vi "ProducerConsumerStyle VI.vi"() -> ()   [LabVIEW 2023]
doc: "Use this template to build a producer/consumer design pattern. Use this template when you need to execute a process, such as data analysis, when a data source, such as a triggered acquisition, produces data at an uneven rate and you need to execute the process when the data becomes available."
uses:
  <vilib>/express/express shared/transition.llb/Dynamic To Waveform Array.vi
  <vilib>/express/express signal manip/GetorSetDDTAttributes/Set DDT Attributes/SetT0.vi
  <vilib>/express/express shared/transition.llb/Waveform Array To Dynamic.vi
  <vilib>/FPGAPlugInAG/USB-7856R OEM/niLvFpga_Open_USB-7856R OEM.vi
  <vilib>/rvi/interface/common/dynamic/niFpgaDynamicAddResources.vi
  <vilib>/rvi/interface/common/niFpgaWaitOnOcc.vi
  <vilib>/Utility/error.llb/Error Cluster From Error Code.vi
  <vilib>/FPGAPlugInAG/Dynamic/niLvFpga_Run_Dynamic.vi
  <vilib>/rvi/errors/niLvFpgaAdjustHostInterfaceError.vi
  <vilib>/FPGAPlugInAG/Dynamic/niLvFpga_Close_Dynamic.vi
  <vilib>/express/express signal manip/GetorSetDDTAttributes/Set DDT Attributes/Set DDT Properties.xnode
  <vilib>/rvi/interface/nirviOpenFPGA/nirviOpenFPGA.xnode
  FPGA Bitfiles/wip_FPGATarget_FPGAVIwithRMS_sDE+ysAwCS4.lvbitx
  FPGA VI with RMS.vi
  <vilib>/rvi/interface/nirviMethod/nirviMethod.xnode
  <vilib>/rvi/interface/nirviReadWriteControl/nirviReadWriteControl.xnode
  <vilib>/rvi/interface/nirviCloseFPGA/nirviCloseFPGA.xnode
  <vilib>/rvi/errors/niLvFpgaMergeErrorWithErrorCode.vi
  <vilib>/FPGAPlugInAG/Dynamic/niLvFpga_ConfigureFifo_Dynamic.vi
  <vilib>/FPGAPlugInAG/Dynamic/niLvFpga_StartFifo_Dynamic.vi
  NiFpgaLv.dll
  <vilib>/rvi/interface/Simulation/niFpgaSimulationCallBeginRW.vi
  <vilib>/FPGAPlugInAG/Dynamic/niLvFpga_ReadFifo_Dynamic.vi
panel:
  out "In Loop timed out?":bool
  out "Saving Data":bool
  in  "Stop Writing Data":bool
  in  "Number of Elements":u32=500
  in  "Count(Ticks)":u32
  out "Elements Remaining":u32
  out "Timed Out?":bool
  out "Loop TIme":u32
  out "Waveform Chart":sgl[](graph)
  out "Actual Depth":u32
  in  "Ending frequency":dbl=32770.0
  in  "Starting frequency":dbl=32750.0
  out "Number of steps":dbl=nan
  out "I/P Frequency Value":dbl
  in  "Step Value":dbl=1.0
  in  "stop":bool
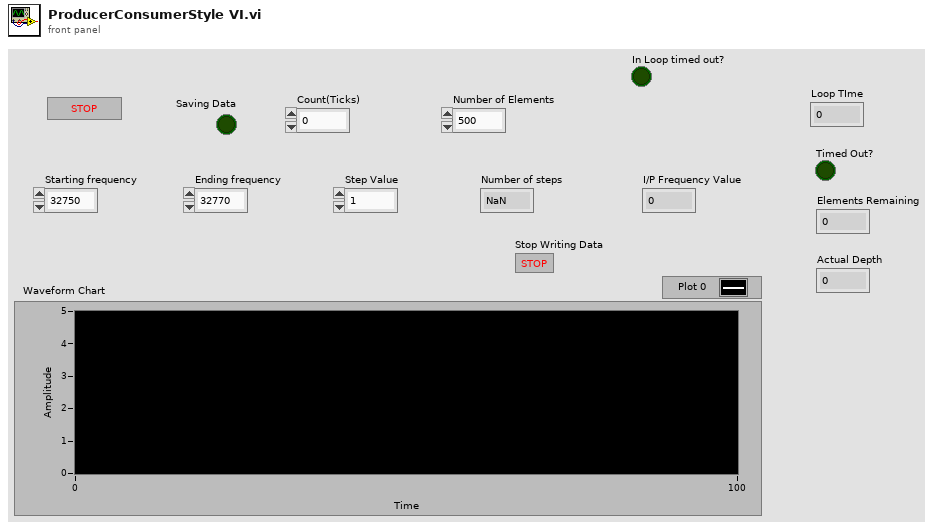
[diagram p1: front panel]
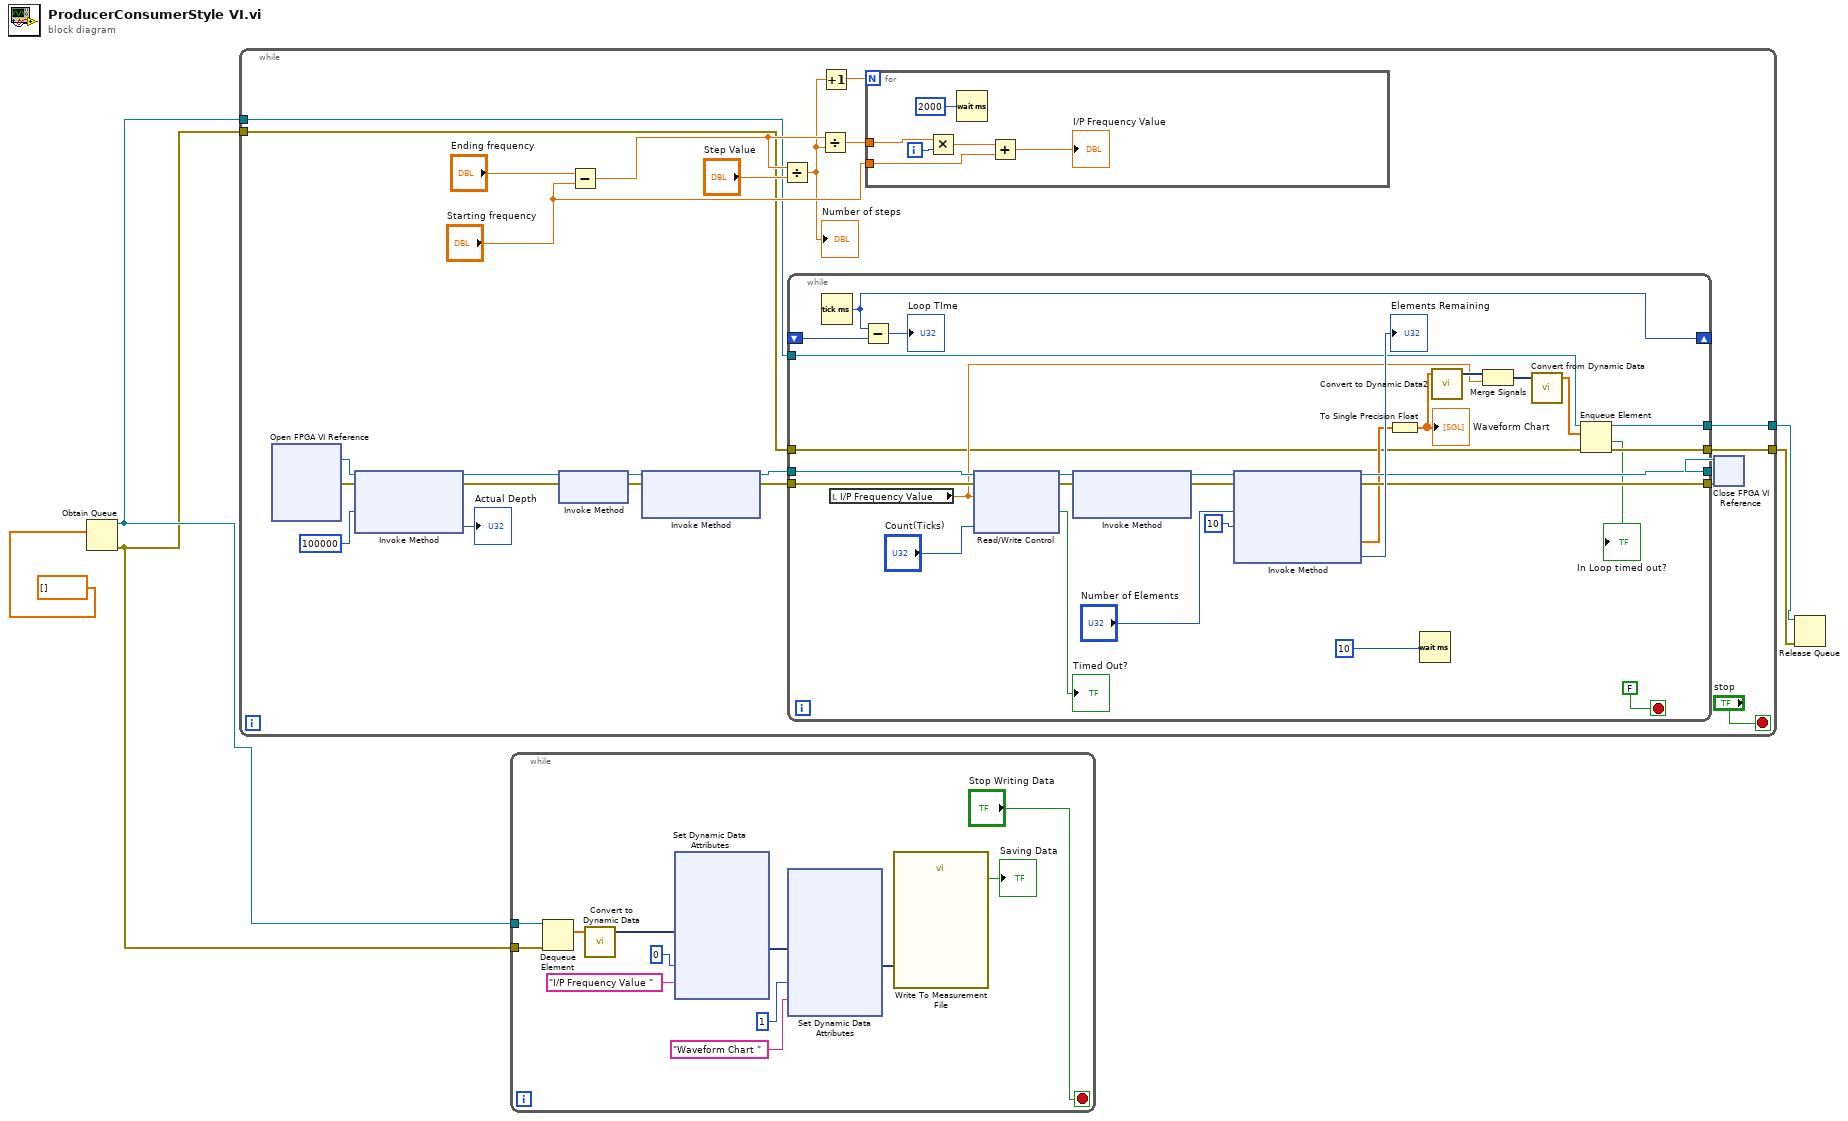
[diagram p0: block diagram]
diagram:
  n1 = Obtain Queue(element data type=dbl[] []) -> (queue out=w2:refnum<queue>, error out=w1:errorcluster)  [unwired: 4 in, 1 out]
  n2 = while {
    tunnel: [w9] -> w5
    tunnel: [w8] -> w4
    tunnel: w2 -> [w7]
    tunnel: w1 -> [w6]
    stop <- "stop" stop-if-true
    n3 = xnode "Open FPGA VI Reference"() -> ("FPGA VI Reference Out"=w28:refnum<k20>, "error out"=w27:errorcluster)  [unwired: 2 in]
    n4 = xnode "Invoke Method"("FPGA VI Reference In"=w28, "error in"=w27, "Requested Depth"=u32 100000) -> ("FPGA VI Reference Out"=w25:refnum<k20>, "error out"=w24:errorcluster, "Actual Depth"=→"Actual Depth":u32)
    n5 = xnode "Invoke Method"("FPGA VI Reference In"=w25, "error in"=w24) -> ("FPGA VI Reference Out"=w20:refnum<k20>, "error out"=w19:errorcluster)
    n6 = Subtract(x="Ending frequency", y="Starting frequency") -> (x-y=w12:dbl)
    n7 = xnode "Invoke Method"("FPGA VI Reference In"=w20, "error in"=w19) -> ("FPGA VI Reference Out"=w17:refnum<k20>, "error out"=w18:errorcluster)  [unwired: 1 in]
    n8 = Divide(x=w12, y="Step Value") -> (x/y=w10:dbl)
    "Number of steps" <- w10
    n9 = while {
      tunnel: [w62] -> w23
      tunnel: [w59] -> w22
      tunnel: w17 -> [w56]
      tunnel: w18 -> [w55]
      shift-right: [w51] -> _
      shift-left: _ -> [w50]
      tunnel: [w41] -> w9
      tunnel: [w40] -> w8
      tunnel: w7 -> [w39]
      tunnel: w6 -> [w38]
      stop <- FALSE stop-if-true
      n10 = Tick Count (ms)() -> (millisecond timer value=w51:u32)
      n11 = local read "I/P Frequency Value"() -> (w45:dbl)
      n12 = Subtract(x=w51, y=w50) -> (x-y=→"Loop TIme":u32)
      n13 = xnode "Read/Write Control"("FPGA VI Reference In"=w56, "error in"=w55, "Frequency"=w45, "Count(Ticks)"="Count(Ticks)") -> ("FPGA VI Reference Out"=w54:refnum<k20>, "error out"=w53:errorcluster, "Timed Out?"=→"Timed Out?":bool)
      n14 = xnode "Invoke Method"("FPGA VI Reference In"=w54, "error in"=w53) -> ("FPGA VI Reference Out"=w58:refnum<k20>, "error out"=w57:errorcluster)  [unwired: 1 in]
      n15 = xnode "Invoke Method"("FPGA VI Reference In"=w58, "error in"=w57, "Number of Elements"="Number of Elements", "Timeout (ms)"=10) -> ("FPGA VI Reference Out"=w62:refnum<k20>, "error out"=w59:errorcluster, "Data"=w48:sgl[], "Elements Remaining"=→"Elements Remaining":u32)
      n16 = To Single Precision Float(number=w48) -> (single precision float=w47:sgl[])
      "Waveform Chart" <- w47
      n17 = Wait (ms)(milliseconds to wait=u32 10) -> ()  [unwired: 1 out]
      n18 = call "Convert to Dynamic Data2"("Array"=w47) -> ("Dynamic Data Type"=w46:dynamicdata)  [unwired: 3 in]
      n19 = Merge Signals(w46, w45) -> (w44:dynamicdata)
      n20 = call "Convert from Dynamic Data"("Dynamic Data Type"=w44) -> ("Array"=w43:dbl[])  [unwired: 3 in]
      n21 = Enqueue Element(queue=w39, element=w43, error in (no error)=w38) -> (queue out=w41:refnum<queue>, timed out?=→"In Loop timed out?":bool, error out=w40:errorcluster)  [unwired: 1 in]
    }
    n22 = Divide(x=w12, y=w10) -> (x/y=w15:dbl)
    n23 = Increment(x=w10) -> (x+1=w13:dbl)
    n24 = for {
      N: w13 -> [_]
      tunnel: w15 -> [w35]
      tunnel: "Starting frequency" -> [w32]
      i -> [w34]
      n25 = Multiply(x=w35, y=w34) -> (x*y=w33:dbl)
      n26 = Wait (ms)(milliseconds to wait=u32 2000) -> ()  [unwired: 1 out]
      n27 = Add(x=w33, y=w32) -> (x+y=→"I/P Frequency Value":dbl)
    }
    n28 = xnode "Close FPGA VI Reference"("FPGA VI Reference In"=w23, "error in"=w22) -> ()  [unwired: 1 out]
  }
  n29 = while {
    tunnel: w1 -> [w66]
    tunnel: w2 -> [w65]
    stop <- "Stop Writing Data" stop-if-true
    n30 = Dequeue Element(queue=w65, error in (no error)=w66) -> (element=w76:dbl[])  [unwired: 1 in, 3 out]
    n31 = call "Convert to Dynamic Data"("Array"=w76) -> ("Dynamic Data Type"=w68:dynamicdata)  [unwired: 3 in]
    n32 = xnode "Set Dynamic Data Attributes"("Signals In"=w68, "Signal Index"=0, "Signal Name"="I/P Frequency Value ") -> ("Signals Out"=w74:dynamicdata)  [unwired: 1 in, 1 out]
    n33 = xnode "Set Dynamic Data Attributes"("Signals In"=w74, "Signal Index"=1, "Signal Name"="Waveform Chart ") -> ("Signals Out"=w69:dynamicdata)  [unwired: 1 in, 1 out]
    n34 = call "Write To Measurement File"("Signals"=w69) -> ("Saving Data"=→"Saving Data":bool)  [unwired: 16 in, 2 out]
  }
  n35 = Release Queue(queue=w5, error in (no error)=w4) -> ()  [unwired: 1 in, 3 out]
